vi "Write Nil.vi"   [LabVIEW 2017, in "LabPack.lvlib" / "Writer.lvclass"]
doc: "Writes and encodes a Nil to the MessagePack binary data format."
uses:
  Writer.lvclass
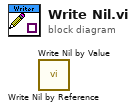
[diagram p0: block diagram]
diagram:
  n1 = call "Write Nil by Reference.vi"() -> ()  [unwired: 10 in, 2 out]
  n2 = call "Write Nil by Value.vi"() -> ()  [unwired: 10 in, 2 out]
